vi "Get Value (U32).vi"(8 "error in":errorcluster, 11 "Sub Obj in":refnum<class "Sub Object.lvclass">) -> (0 "error out":errorcluster, 2 "Value":u32, 3 "Sub Obj out":refnum<class "Sub Object.lvclass">)   [LabVIEW 2020, in "CANopen.lvlib" / "Sub Object.lvclass"]
uses:
  Sub Object.lvclass
  Sub Object.lvclass/Sub Object.ctl
  CANopen.lvlib
  Typedefs/Data Type.ctl
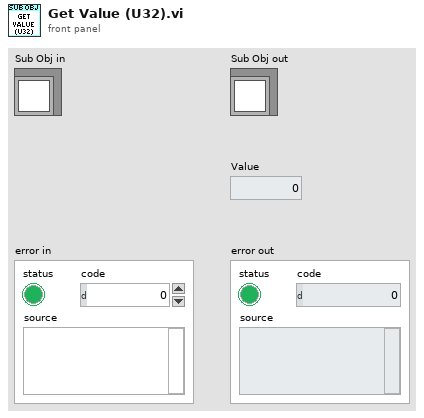
[diagram p1: front panel]
types:
  T1 = typedef "CANopen.lvlib/Data Type.ctl" = u16
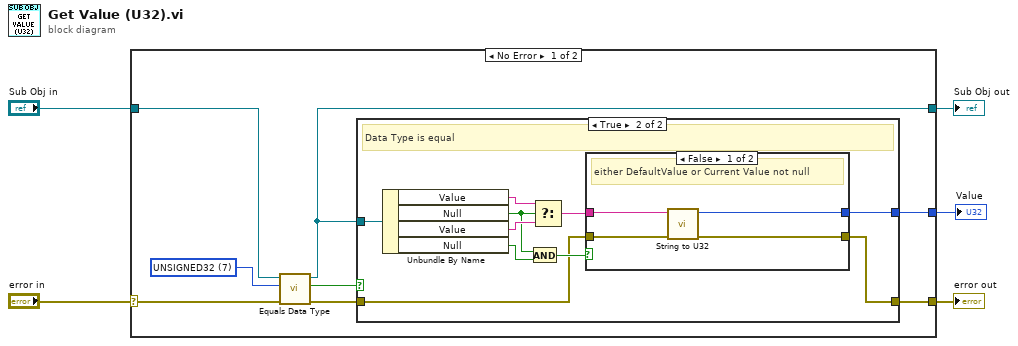
[diagram p0: block diagram]
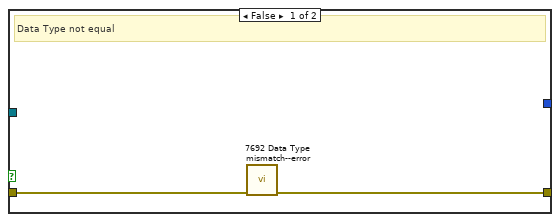
[diagram p2: hidden frame]
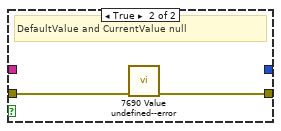
[diagram p3: hidden frame]
diagram:
  n1 = case shown="No Error" "error in" {
    selector: "error in" -> [w13 w33]
    tunnel: [w12 w33] -> w2
    tunnel: [w8 w32] -> w4
    tunnel: "Sub Obj in" -> [w9 w32]
    tunnel: [w11 _] -> w1
    frame No Error {
      w6 = T1 7 items=["BOOLEAN"=1, "INTEGER8"=2, "INTEGER16"=3, "INTEGER32"=4, "UNSIGNED8"=5, "UNSIGNED16"=6, "UNSIGNED32"=7, "REAL32"=8, "VISIBLE_STRING"=9, "OCTET_STRING"=10, "UNICODE_STRING"=11, "TIME_OF_DAY"=12, "TIME_DIFFERENCE"=13, "RESERVED1"=14, "DOMAIN"=15, "INTEGER24"=16, "REAL64"=17, "INTEGER40"=18, "INTEGER48"=19, "INTEGER56"=20, "INTEGER64"=21, "UNSIGNED24"=22, "RESERVED2"=23, "UNSIGNED40"=24, "UNSIGNED48"=25, "UNSIGNED56"=26, "UNSIGNED64"=27, "RESERVED3"=28, "RESERVED4"=29, "RESERVED5"=30, "RESERVED6"=31, "PDO_COMMUNICATION_PARAMETER"=32, "PDO_MAPPING"=33, "SDO_PARAMETER"=34, "IDENTITY"=35, "RESERVED7"=36] ("Data Type")
      n2 = call "Equals Data Type.vi"("error in"=w13, "Data Type"=w6, "Sub Obj in"=w9) -> ("error out"=w10:errorcluster, "Equal"=w7:bool, "Sub Obj out"=w8:refnum<class "Sub Object.lvclass">)  [unwired: 6 in]
      n3 = case shown="True" w7 {
        tunnel: [w14 w25] -> w12
        tunnel: [_ w18] -> w11
        tunnel: w8 -> [_ w16]
        tunnel: w10 -> [w15 w17]
        frame False {
          # "Data Type not equal"
          n4 = call "7692 Data Type mismatch--error.vi"("error in"=w15) -> ("error out"=w14:errorcluster)  [unwired: 9 in, 1 out]
        }
        frame True {
          # "Data Type is equal"
          n5 = Unbundle By Name(w16) -> ("Value"=w24:string, "Null"=w20:bool, "Value"=w22:string, "Null"=w21:bool)
          n6 = And(x=w20, y=w21) -> (x .and. y?=w19:bool)
          n7 = Select(t=w24, s=w20, f=w22) -> (s? t:f=w23:string)
          n8 = case shown="False" w19 {
            tunnel: w17 -> [w28 w31]
            tunnel: [w27 w30] -> w25
            tunnel: w23 -> [w29 _]
            tunnel: [w26 _] -> w18
            frame False {
              # "either DefaultValue or Current Value not null"
              n9 = call "String to U32.vi"("error in"=w28, "Integer String"=w29) -> ("error out"=w27:errorcluster, "U32"=w26:u32)  [unwired: 8 in]
            }
            frame True {
              # "DefaultValue and CurrentValue null"
              n10 = call "7690 Value undefined--error.vi"("error in"=w31) -> ("error out"=w30:errorcluster)  [unwired: 9 in, 1 out]
            }
          }
        }
      }
    }
    frame Error {
    }
  }
  "Sub Obj out" <- w4
  "error out" <- w2
  "Value" <- w1
